vi "Debug Message Loop.vi"(8 "error in (no error)":errorcluster, 11 "Refnum in":refnum<k33>) -> (0 "error out":errorcluster)   [LabVIEW 2020]
uses:
  Console Message Type.ctl
  Waveform Analog Output Engine.lvlib
  <vilib>/NI VeriStand/Custom Device Tools/Custom Device Utility Library/Custom Device Utility Library.lvlib
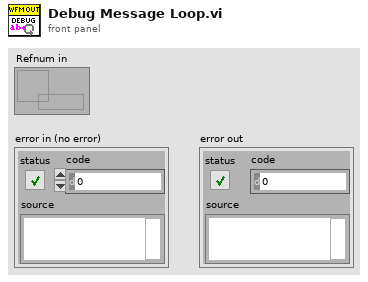
[diagram p1: front panel]
types:
  T1 = typedef "Waveform Analog Output Engine.lvlib/Console Message Type.ctl" = enum16{"Range Warning", "Error"}
  T2 = cluster{"Hw Max":dbl, "Hw Min":dbl, "Requested Amplitude":dbl, "Requested Offset":dbl, "Coerced Amplitude":dbl, "Coerced Offset":dbl}
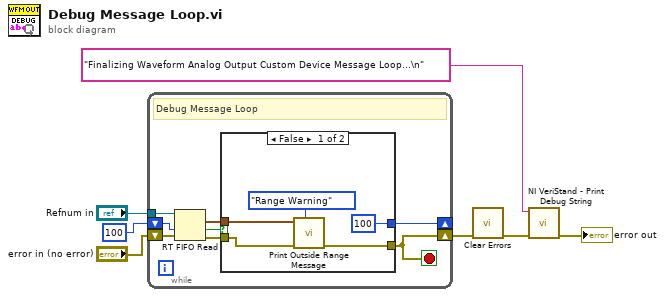
[diagram p0: block diagram]
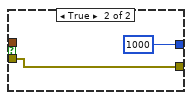
[diagram p2: hidden frame]
diagram:
  n1 = while "Debug Message Loop" {
    tunnel: "Refnum in" -> [w14]
    shift-right: [w10] -> w5
    shift-left: "error in (no error)" -> [w15]
    shift-right: [w9] -> _
    shift-left: 100 ("milliseconds to wait") -> [w8]
    stop <- w10 stop-if-true
    # "Debug Message Loop"
    n2 = RT FIFO Read(0:w14, 2:w8, 3:w15) -> (9:w12:T2, 10:w13:bool, 11:w11:errorcluster)  [unwired: 1 in, 2 out]
    n3 = case shown="False" w13 {
      tunnel: w12 -> [w18 _]
      tunnel: w11 -> [w17 w21]
      tunnel: [w17 w21] -> w10
      tunnel: [100 ("milliseconds to wait") 1000 ("milliseconds to wait")] -> w9
      frame False {
        n4 = call "Print Outside Range Message.vi"("Message Type"=Console_Message_Type."Range Warning", "error in (no error)"=w17, "Message Values"=w18) -> ()  [unwired: 9 in]
      }
      frame True {
      }
    }
  }
  n5 = call <vilib>:"Clear Errors.vi"("error in (no error)"=w5) -> ("error out"=w4:errorcluster)  [unwired: 5 in, 1 out]
  n6 = call <vilib>:"NI VeriStand - Print Debug String.vi"("error in (no error)"=w4, "Message"="Finalizing Waveform Analog Output Custom Device Message Loop...\n") -> ("error out"=→"error out":errorcluster)  [unwired: 9 in]
